vi "X Array Range to Index.vi"(2 "X Range":dbl, 3 "X-array":dbl[](array[numeric])) -> (0 "X Range (index)":i32)   [LabVIEW 2019, in "xy_utilities.lvlib"]
uses:
  xy_utilities.lvlib
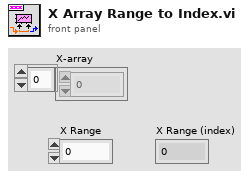
[diagram p1: front panel]
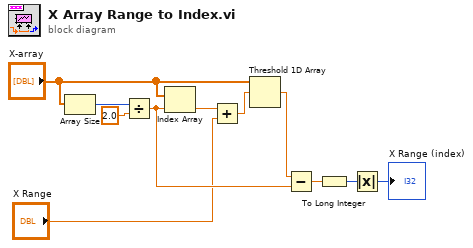
[diagram p0: block diagram]
diagram:
  n1 = Array Size(array="X-array") -> (size(s)=w1:i32)
  n2 = Divide(x=w1, y=2.0) -> (x/y=w10:dbl)
  n3 = Index Array(array="X-array", index=w10) -> (element=w3:dbl)
  n4 = Add(x=w3, y="X Range") -> (x+y=w5:dbl)
  n5 = Threshold 1D Array(2:w5, 3:"X-array") -> (0:w9:dbl)  [unwired: 1 in]
  n6 = Subtract(x=w9, y=w10) -> (x-y=w4:dbl)
  n7 = To Long Integer(number=w4) -> (32bit integer=w6:i32)
  n8 = Absolute Value(x=w6) -> (abs(x)=→"X Range (index)":i32)
